vi "select spot when imaging.vi"(10 "current location":T3, 11 "spot location constraints":T4=[{"spot number"=0, "active"=FALSE, "x max"=0, "x min"=0, "y max"=0, "y min"=0}, {"spot number"=0, "active"=FALSE, "x max"=0, "x min"=0, "y max"=0, "y min"=0}, {"spot number"=0, "active"=FALSE, "x max"=0, "x min"=0, "y max"=0, "y min"=0}, {"spot number"=0, "active"=FALSE, "x max"=0, "x min"=0, "y max"=0, "y min"=0}]) -> (0 "update tracking?":T1, 1 "use photons to track":bool, 3 "selected spot":T2)   [LabVIEW 2010]
uses:
  spot location constraints.ctl
  spot location constraint.ctl
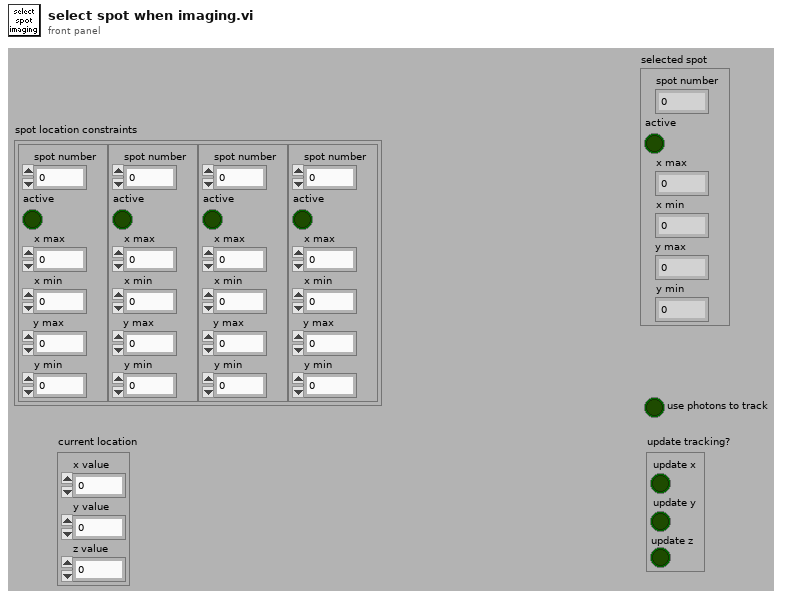
[diagram p1: front panel]
types:
  T1 = cluster{"update x":bool, "update y":bool, "update z":bool}
  T2 = typedef "spot location constraint.ctl" = cluster{"spot number":i8, "active":bool, "x max":i16, "x min":i16, "y max":i16, "y min":i16}
  T3 = cluster{"x value":i16, "y value":i16, "z value":i16}
  T4 = typedef "spot location constraints.ctl" = T2[]
  T5 = cluster{"crossing":bool, "crossing":bool, "crossing":bool}
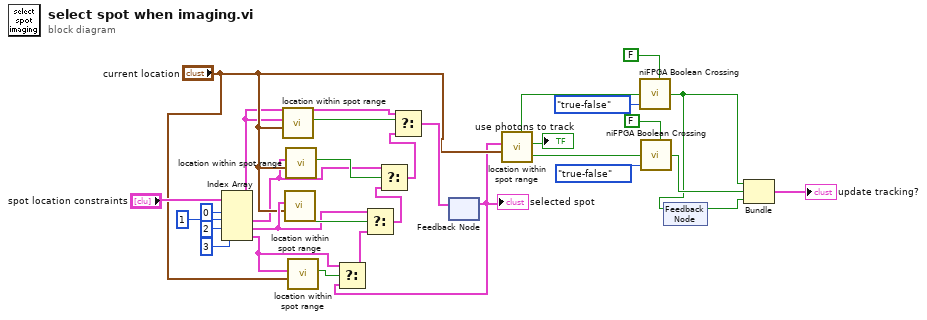
[diagram p0: block diagram]
diagram:
  n1 = Index Array(array="spot location constraints", index #1=0 ("index"), index #2=1 ("index"), index #3=2 ("index"), index #4=3 ("index")) -> (element #1=w2:T2, element #2=w1:T2, element #3=w21:T2, element #4=w24:T2)
  n2 = call "location within spot range"("current location"="current location", "spot location constraint"=w2) -> ("spot selected"=w17:bool)  [unwired: 7 in, 2 out]
  n3 = call "location within spot range"("current location"="current location", "spot location constraint"=w21) -> ("spot selected"=w22:bool)  [unwired: 7 in, 2 out]
  n4 = call "location within spot range"("current location"="current location", "spot location constraint"=w1) -> ("spot selected"=w20:bool)  [unwired: 7 in, 2 out]
  n5 = call "location within spot range"("current location"="current location", "spot location constraint"=w24) -> ("spot selected"=w25:bool)  [unwired: 7 in, 2 out]
  n6 = feedback #1() -> (w10:T2)  [unwired: 1 in]
  "selected spot" <- w10
  n7 = Select(t=w24, s=w25, f=w10) -> (s? t:f=w23:T2)
  n8 = Select(t=w21, s=w22, f=w23) -> (s? t:f=w19:T2)
  n9 = Select(t=w1, s=w20, f=w19) -> (s? t:f=w18:T2)
  n10 = Select(t=w2, s=w17, f=w18) -> (s? t:f=w16:T2)
  n11 = feedback-in #1(w16) -> ()
  n12 = call "location within spot range"("current location"="current location", "spot location constraint"=w10) -> ("spot selected"=→"use photons to track":bool, "y-valid"=w9:bool, "x-valid"=w13:bool)  [unwired: 7 in]
  n13 = call <vilib>:"niFPGA Boolean Crossing.vi"("input"=w13, "direction"=enum8{"either", "false-true", "true-false"}."true-false", "initialize"=FALSE) -> ("crossing"=w4:bool)  [unwired: 6 in]
  n14 = call <vilib>:"niFPGA Boolean Crossing.vi"("input"=w9, "direction"=enum8{"either", "false-true", "true-false"}."true-false", "initialize"=FALSE) -> ("crossing"=w5:bool)  [unwired: 6 in]
  n15 = feedback-in #2(w4) -> ()
  n16 = feedback #2() -> (w6:bool)  [unwired: 1 in]
  n17 = Bundle("crossing"=w4, "crossing"=w5, "crossing"=w6) -> (→"update tracking?":T5)  [unwired: 1 in]
